vi "NF87XX.connect.vi"(0 "i ref in":refnum<vi>, 2 "Connect?":bool, 5 "error in (no error)":errorcluster) -> (14 "i ref out":refnum<vi>, 19 "error out":errorcluster)   [LabVIEW 2014, in "NF87XX.lvlib"]
doc: "Depending on a naming convention, this VI opens a VISA session or a TCPIP connection to the controller if \"Connect?\" is true, otherwise the session is closed. If true is chosen, it saves the connection related data also to own attributes for further use. \n\nauthor: Stefan Götte\ndata: 30-AUG-2006\n\n\nLicense Agreement for this software:\n\nCopyright (C)\nGesellschaft für Schwerionenforschung, GSI\nPlanckstr. 1\n64291 Darmstadt\nGermany\n\nContact: D.Beck@gsi.de \n\nThis program is free software; you can redistribute it and/or modify it under the terms of the GNU General Public License as published by the Free Software Foundation; either version 2 of the license, or (at your option) any later version.\n\nThis program is distributed in the hope that it will be useful, but WITHOUT ANY WARRANTY; without even the implied warranty of MERCHANTABILITY or FITNESS FOR A PARTICULAR PURPOSE. See the GNU General License for more details (http://www.gnu.org).\n\nGesellschaft für Schwerionenforschung, GSI\nPlanckstr. 1, 64291 Darmstadt, Germany\nFor all questions and ideas contact: M.Richter@gsi.de, H.Brand@gsi.de or D.Beck@gsi.de.\nLast update: 17-JUN-2004"
uses:
  NF87XX.lvlib
  non_GPL/instr.lib/NewFocusPico/VISA & TCPIP Control.ctl
  non_GPL/instr.lib/NewFocusPico/MCL Cmd Cluster.ctl
  non_GPL/instr.lib/NewFocusPico/NewFocusPico - Driver np.lvlib
panel:
  in  "Con Sets":T1={"VISA or TCP/IP"=FALSE, "Init Connection"=TRUE, "Close Connection"=FALSE, "Resource Name"="COM1", "hostname"="N/A", "connection ID"=refnum}
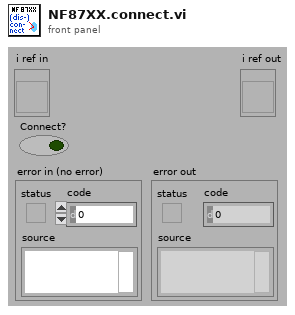
[diagram p1: front panel]
types:
  T1 = typedef "NewFocusPico - Driver np.lvlib/VISA & TCPIP Control.ctl" = cluster{"VISA or TCP/IP":bool, "Init Connection":bool, "Close Connection":bool, "Resource Name":refnum<visa-resource-name>, "hostname":string, "connection ID":refnum<k5>}
  T2 = typedef "NewFocusPico - Driver np.lvlib/MCL Cmd Cluster.ctl" = cluster{"MCL Cmd":enum16{"User....", "DEF", "DIAG", "INI", "LOCK", "UNLOCK", "MAP", "SAV", "VER", "ACC", "CHL", "FOR", "GO", "HAL", "MOF", "MON", "MPV", "POS", "REL", "REV", "STA", "STO", "TYP", "VEL", "ABS", "SER", "NOS", "DRT", "FLI", "RLI", "FIN", "RIN", "AIN", "IN", "JOF", "JON", "OUT", "RES FINE", "RES COARSE", "02 (HEX)", "PWM", "CNT", "TMR", "HOSTNAME", "IPADDR", "IPMODE", "NETMASK", "GATEWAY", "DNSSRVR", "PASSWD", "ECHO", "MACADDR"}, "User Cmd/Numeric Argu":string, "Query/Set":enum16{"Query", "Set"}}
  T3 = typedef "NF87XX.lvlib/NF87XX.i attribute.ctl" = cluster{"Con Settings":T1, "Drivers":T4[], "Status":cluster{"Service ID":i32, "Status":T7}, "Joystick available":bool, "VISA Resource":string}
  T4 = typedef "NF87XX.lvlib/NF87XX.driver Settings.ctl" = cluster{"Name":string, "Driver Type":T5, "Pico Parameter type":T6, "Acceleration [Steps/s²]":cluster{"Motor 0":dbl, "Motor 1":dbl, "Motor 2":dbl}, "Start Velocity [Steps/s]":cluster{"Motor 0":dbl, "Motor 1":dbl, "Motor 2":dbl}, "Velocity [Steps/s]":cluster{"Motor 0":dbl, "Motor 1":dbl, "Motor 2":dbl}, "axis channel":i32, "Position":i32, "Position Service ID":i32}
  T5 = typedef "NF87XX.lvlib/NF87XX.driver Type.ctl" = enum16{"not defined", "3-ch open loop drv", "1-ch closed loop drv"}
  T6 = typedef "NewFocusPico - Driver np.lvlib/Pico Parameters.ctl" = cluster{"Pico Type":enum16{"Open-Loop Pico", "Close-Loop Pico", "Pico Ultra"}, "Acceleration (steps/sec^2)":string, "Velocity ( Hz)":string, "Driver":string, "Motor":string, "Channel":string, "Process Step":string}
  T7 = typedef "PH_StatusHandler.lvlib/PH_StatusHandler.Status.ctl" = i16
  T8 = typedef "NewFocusPico - Driver np.lvlib/Error.ctl" = errorcluster
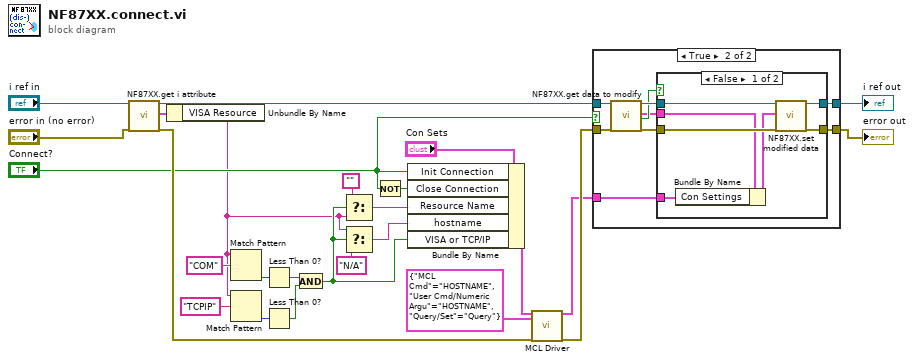
[diagram p0: block diagram]
diagram:
  n1 = call "NF87XX.get i attribute.vi"("i ref in"="i ref in", "error in (no error)"="error in (no error)") -> ("i ref out"=w22:refnum<vi>, "i attribute"=w3:T3, "error out"=w12:errorcluster)  [unwired: 15 in]
  n2 = Unbundle By Name(w3) -> ("VISA Resource"=w1:string)
  n3 = Match Pattern(string=w1, regular expression="COM") -> (offset past match=w17:i32)  [unwired: 1 in, 3 out]
  n4 = Match Pattern(string=w1, regular expression="TCPIP") -> (offset past match=w16:i32)  [unwired: 1 in, 3 out]
  n5 = Less Than 0?(x=w17) -> (x < 0?=w13:bool)
  n6 = Less Than 0?(x=w16) -> (x < 0?=w14:bool)
  n7 = And(x=w13, y=w14) -> (x .and. y?=w4:bool)
  n8 = Select(t="", s=w4, f=w1) -> (s? t:f=w9:string)
  n9 = Select(t=w1, s=w4, f="N/A") -> (s? t:f=w5:string)
  n10 = Not(x="Connect?") -> (.not. x?=w7:bool)
  n11 = Bundle By Name(cluster="Con Sets", "Init Connection"="Connect?", "Close Connection"=w7, "Resource Name"=w9, "hostname"=w5, "VISA or TCP/IP"=w4) -> (w23:T1)
  n12 = call "MCL Driver.vi"("Con Sets in"=w23, "MCL Command"=T2 {"MCL Cmd"=enum."HOSTNAME", "User Cmd/Numeric Argu"="HOSTNAME", "Query/Set"=enum."Query"}, "Error In (no error)"=w12) -> ("Con Sets out"=w10:T1, "Error Out"=w20:T8)  [unwired: 12 in, 3 out]
  n13 = case shown="True" "Connect?" {
    tunnel: w22 -> [w28 w36]
    tunnel: [w28 w35] -> w21
    tunnel: w20 -> [w27 w33]
    tunnel: [w27 w32] -> w19
    tunnel: w10 -> [_ w29]
    frame False {
    }
    frame True {
      n14 = call "NF87XX.get data to modify.vi"("i ref in"=w36, "error in (no error)"=w33) -> ("i ref out"=w37:refnum<vi>, "i attribute"=w30:T3, "timed out"=w31:bool, "error out"=w34:errorcluster)  [unwired: 14 in]
      n15 = case shown="False" w31 {
        tunnel: w37 -> [w44 w46]
        tunnel: [w43 w46] -> w35
        tunnel: w34 -> [w42 w45]
        tunnel: [w41 w45] -> w32
        tunnel: w30 -> [w40 _]
        tunnel: w29 -> [w39 _]
        frame False {
          n16 = Bundle By Name(cluster=w40, "Con Settings"=w39) -> (w38:T3)
          n17 = call "NF87XX.set modified data.vi"("i ref in"=w44, "i attribute"=w38, "error in (no error)"=w42) -> ("i ref out"=w43:refnum<vi>, "error out"=w41:errorcluster)  [unwired: 15 in]
        }
        frame True {
        }
      }
    }
  }
  "error out" <- w19
  "i ref out" <- w21
